vi "I2C error.vi"(10 "return":i32, 11 "error in":errorcluster) -> (3 "error out":errorcluster)   [LabVIEW 2017]
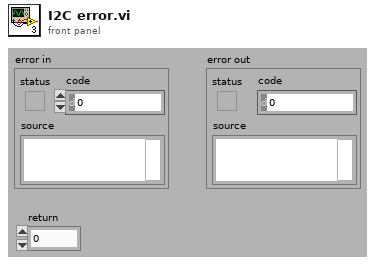
[diagram p1: front panel]
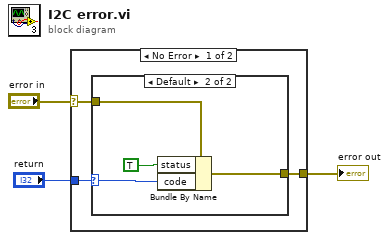
[diagram p0: block diagram]
diagram:
  n1 = case shown="No Error" "error in" {
    selector: "error in" -> [w4 w12]
    tunnel: [w5 w12] -> w3
    tunnel: "return" -> [w6 _]
    frame No Error {
      n2 = case shown="Default" w6 {
        selector: w6 -> [_ w9]
        tunnel: [w7 w10] -> w5
        tunnel: w4 -> [w7 w11]
        frame 0 {
        }
        frame Default {
          n3 = Bundle By Name(cluster=w11, "status"=TRUE, "code"=w9) -> (w10:errorcluster)
        }
      }
    }
    frame Error {
    }
  }
  "error out" <- w3
